vi "读取CODMn数据波形新.vi"() -> ()   [LabVIEW 2016, in "斯坦道CODMn新电路板.lvlib"]
uses:
  <vilib>/Utility/miscctls.llb/LVPointTypeDef.ctl
  <userlib>/_OpenG.lib/array/array.llb/Sort 1D Array (I32)__ogtk.vi
  <vilib>/Waveform/WDTFileIO.llb/Read Waveform from File.vi
panel:
  in  "页":i32 format="第%.0f页"
  in  "每页条数":i32=20
  in  "向后按钮":bool
  in  "向前按钮":bool
  in  "数据表":T1
  in  "查看曲线数组":bool[](array[boolean])
  in  "打开波形文件":bool
  in  "簇":cluster{"数据起始时间":timestamp, "数据终止时间":timestamp}
  in  "查询":bool
  in  "当前滴定曲线":bool
  in  "当前温度曲线":bool
  in  "关闭":bool
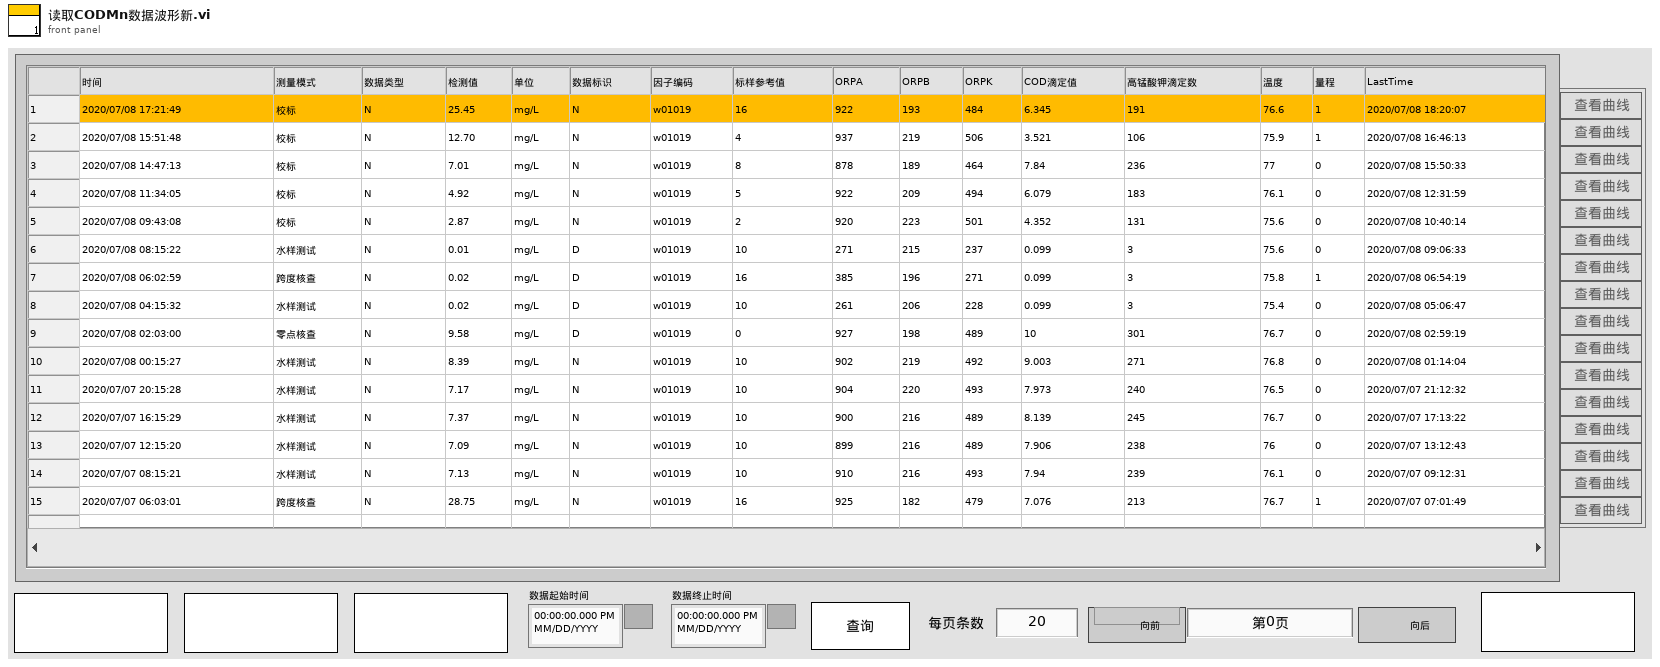
[diagram p1: front panel]
types:
  T1 = typedef "数据查询大列表框.ctl" = i32
  T2 = typedef "LVPointTypeDef.ctl" = cluster{"Horizontal":i16, "Vertical":i16}
  T3 = cluster{timestamp, "seconds since 1Jan1904":timestamp}
  T4 = enum16{"Left Button", "Center Button", "Right Button", "Window Close"}
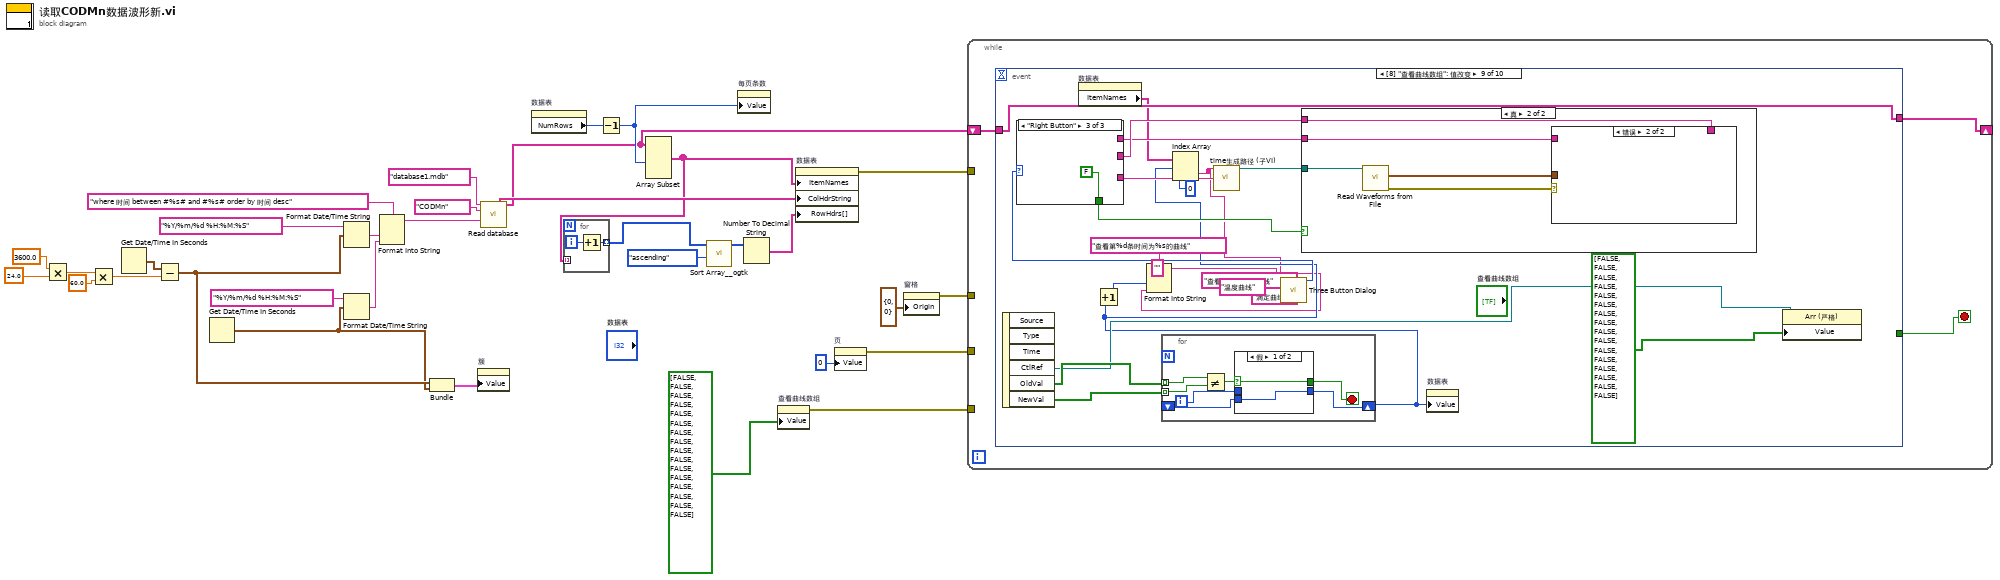
[diagram p0: block diagram]
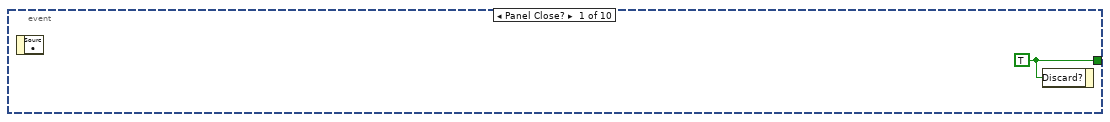
[diagram p2: hidden frame]
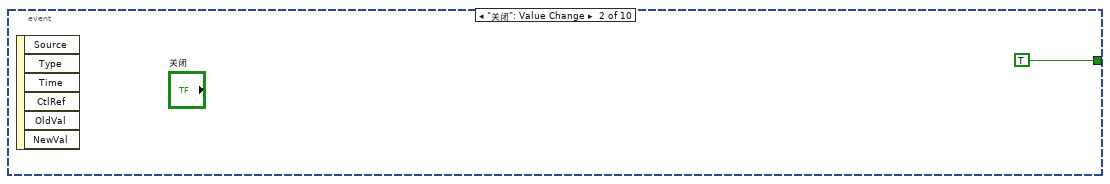
[diagram p3: hidden frame]
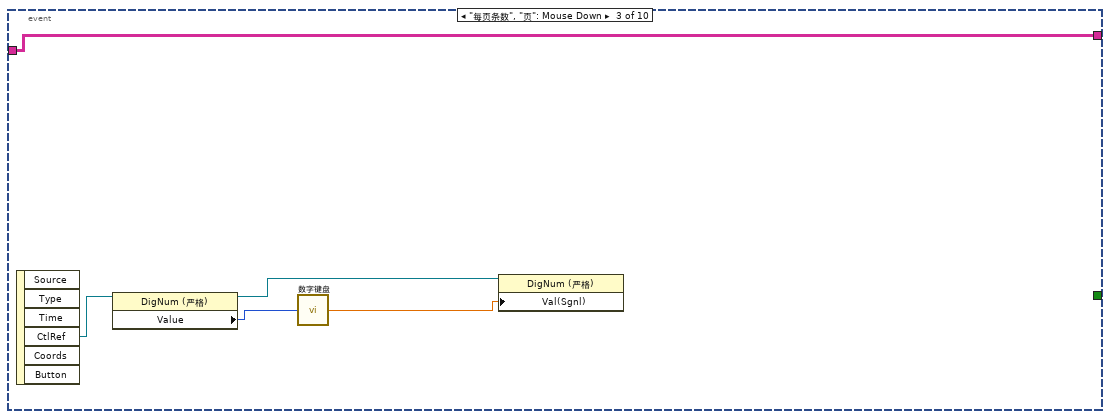
[diagram p4: hidden frame]
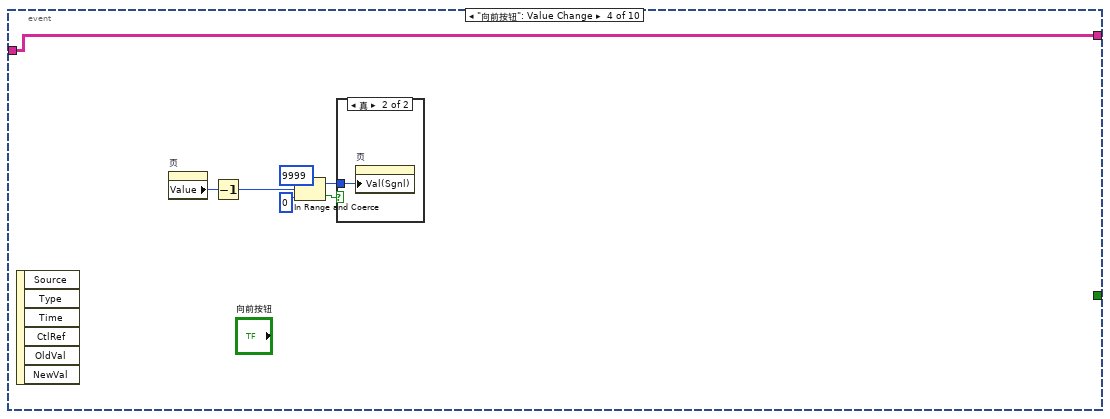
[diagram p5: hidden frame]
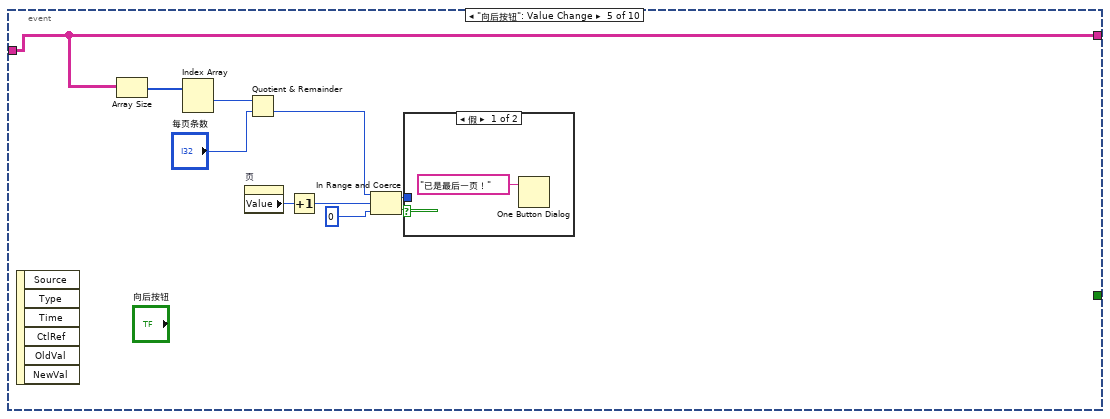
[diagram p7: hidden frame]
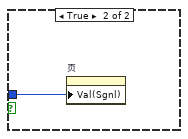
[diagram p8: hidden frame]
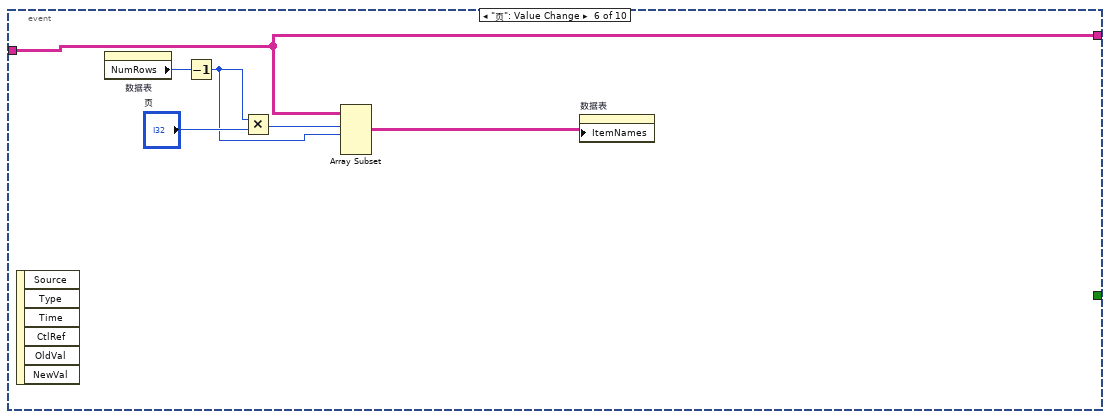
[diagram p9: hidden frame]
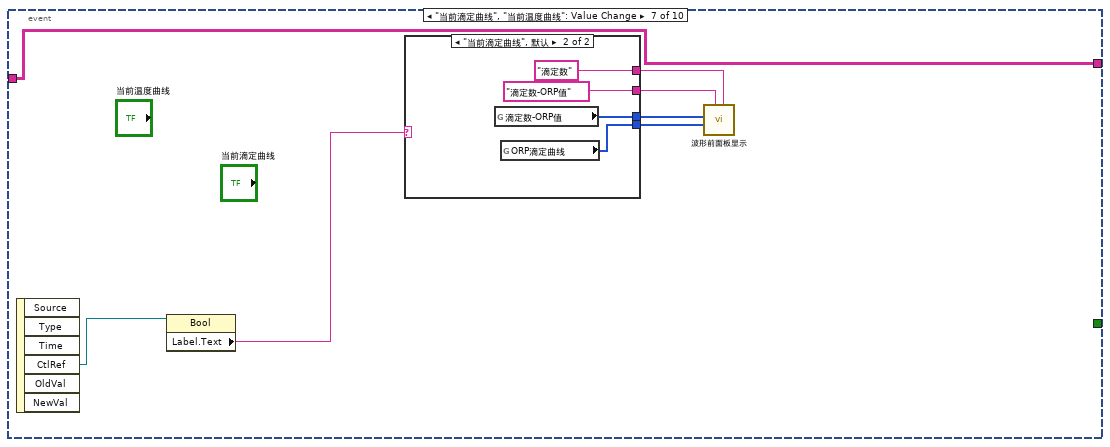
[diagram p10: hidden frame]
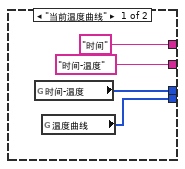
[diagram p11: hidden frame]
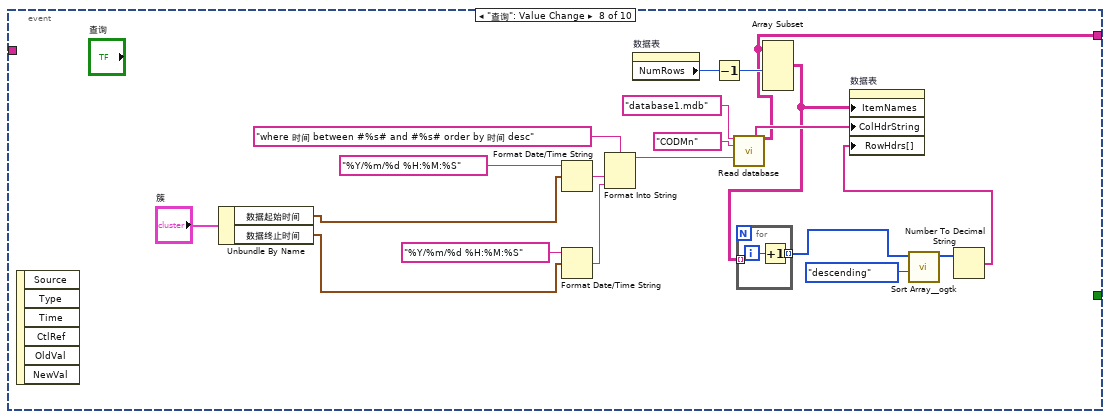
[diagram p12: hidden frame]
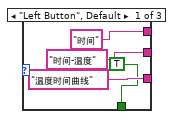
[diagram p14: hidden frame]
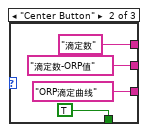
[diagram p15: hidden frame]
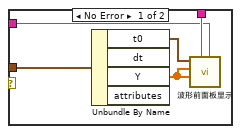
[diagram p17: hidden frame]
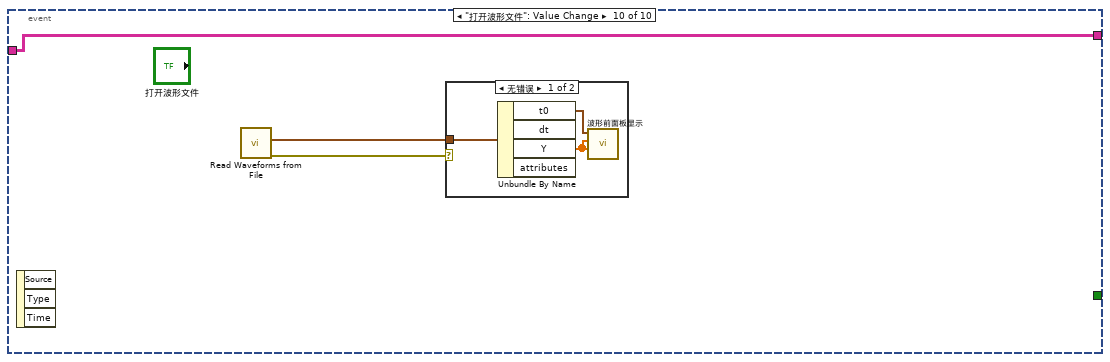
[diagram p18: hidden frame]
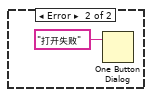
[diagram p19: hidden frame]
diagram:
  n1 = Multiply(x=3600.0, y=24.0) -> (x*y=w30:dbl)
  n2 = Multiply(x=w30, y=60.0) -> (x*y=w28:dbl)
  n3 = Get Date/Time In Seconds() -> (seconds since 1Jan1904=w33:timestamp)
  n4 = Subtract(x=w33, y=w28) -> (x-y=w3:timestamp)
  n5 = Get Date/Time In Seconds() -> (seconds since 1Jan1904=w2:timestamp)
  n6 = Format Date/Time String(time format string (%c)="%Y/%m/%d %H:%M:%S" ("时间格式字符串(%c)"), seconds (now)=w3) -> (date/time string=w25:string)  [unwired: 1 in]
  n7 = Format Date/Time String(time format string (%c)="%Y/%m/%d %H:%M:%S" ("时间格式字符串(%c)"), seconds (now)=w2) -> (date/time string=w26:string)  [unwired: 1 in]
  n8 = Format Into String(format string="where 时间 between #%s# and #%s# order by 时间 desc" ("condition"), w25, w26) -> (resulting string=w27:string)  [unwired: 2 in, 1 out]
  n9 = Bundle(w3, "seconds since 1Jan1904"=w2) -> (w1:T3)  [unwired: 1 in]
  n10 = property on="簇" class="Clust (严格)"("Value"=w1) -> ()  [unwired: 2 in, 2 out]
  n11 = call "Read database.vi"("database"="database1.mdb", "组合框"="CODMn", "condition"=w27) -> ("columns"=w19:string[], "表格"=w10:string[][])  [unwired: 7 in, 4 out]
  n12 = property on="数据表" class="MCListbox (严格)"() -> ("NumRows"=w13:u32)  [unwired: 2 in, 2 out]
  n13 = Decrement(x=w13) -> (x-1=w11:u32)
  n14 = Array Subset(array=w10, length (row)=w11) -> (w12:string[][])  [unwired: 3 in]
  n15 = for {
    tunnel: [w34] -> w18 mode=indexing
    tunnel: w12 -> [_] mode=indexing
    i -> [w35]
    n16 = Increment(x=w35) -> (x+1=w34:i32)
  }
  n17 = call-poly <userlib>:"Sort Array__ogtk.vi"("Order"=enum16{"ascending", "descending"}."ascending", "Array in"=w18) -> ("Sorted Array out"=w16:i32[])  [unwired: 8 in, 1 out]
  n18 = property on="每页条数" class="DigNum (严格)"("Value"=w11) -> ()  [unwired: 2 in, 2 out]
  n19 = Number To Decimal String(number=w16) -> (decimal integer string=w15:string[])  [unwired: 1 in]
  n20 = property on="查看曲线数组" class="Arr (严格)"("Value"=bool[] [FALSE, FALSE, FALSE, FALSE, FALSE, FALSE, FALSE, FALSE, FALSE, FALSE, FALSE, FALSE, FALSE, FALSE, FALSE, FALSE] ("查看曲线数组")) -> (error out=w4:errorcluster)  [unwired: 2 in, 1 out]
  n21 = property on="数据表" class="MCListbox (严格)"("ItemNames"=w12, "ColHdrString"=w19, "RowHdrs[]"=w15) -> (error out=w14:errorcluster)  [unwired: 2 in, 1 out]
  n22 = property on="页" class="DigNum (严格)"("Value"=0 ("页")) -> (error out=w8:errorcluster)  [unwired: 2 in, 1 out]
  n23 = property on="窗格" class="Pane"("Origin"=T2 {"Horizontal"=0, "Vertical"=0} ("原点")) -> (error out=w6:errorcluster)  [unwired: 2 in, 1 out]
  n24 = while {
    tunnel: w14 -> [_]
    shift-right: [w36] -> _
    shift-left: w10 -> [w37]
    tunnel: w8 -> [_]
    tunnel: w6 -> [_]
    tunnel: w4 -> [_]
    stop <- w38 stop-if-true
    n25 = event shown="[8] \"查看曲线数组\": 值改变" {
      selector: _ -> [_ _ _ _ _ _ _ _ _ _]
      dyn-events: _ -> [_ _ _ _ _ _ _ _ _ _]
      timeout: _ -> [_ _ _ _ _ _ _ _ _ _]
      tunnel: [w39 TRUE ("Discard?") _ _ _ _ _ _ _ _] -> w38
      tunnel: w37 -> [_ _ w41 w46 w58 w66 w72 _ w113 w160]
      tunnel: [_ _ w41 w46 w58 w66 w72 w87 w113 w160] -> w36
      event Panel Close? {
        w39 = TRUE ("Discard?")
        n26 = event-data() -> ()  [unwired: 1 in, 1 out]
        n27 = event-data("Discard?"=w39) -> ()  [unwired: 1 in, 1 out]
      }
      event "关闭": Value Change {
        n28 = event-data() -> ()  [unwired: 1 in, 6 out]
      }
      event "每页条数", "页": Mouse Down {
        n29 = event-data() -> ("CtlRef"=w45:refnum<vi>)  [unwired: 1 in, 5 out]
        n30 = property class="DigNum (严格)"(reference=w45) -> (reference out=w43:refnum<vi>, "Value"=w44:i32)  [unwired: 1 in, 1 out]
        n31 = call "数字键盘.vi"("OldNumber"=w44) -> ("NewNumber"=w42:dbl)
        n32 = property class="DigNum (严格)"(reference=w43, "Val(Sgnl)"=w42) -> ()  [unwired: 1 in, 2 out]
      }
      event "向前按钮": Value Change {
        n33 = event-data() -> ()  [unwired: 1 in, 6 out]
        n34 = property on="页" class="DigNum (严格)"() -> ("Value"=w47:i32)  [unwired: 2 in, 2 out]
        n35 = Decrement(x=w47) -> (x-1=w52:i32)
        n36 = In Range and Coerce(upper limit=9999 ("上限"), x=w52, lower limit=0 ("下限")) -> (coerced(x)=w49:i32, In Range?=w48:bool)
        n37 = case shown="真" w48 {
          tunnel: w49 -> [_ w53]
          frame False {
          }
          frame True {
            n38 = property on="页" class="DigNum (严格)"("Val(Sgnl)"=w53) -> ()  [unwired: 2 in, 2 out]
          }
        }
      }
      event "向后按钮": Value Change {
        n39 = event-data() -> ()  [unwired: 1 in, 6 out]
        n40 = Array Size(array=w58) -> (size(s)=w57:i32[])
        n41 = Index Array(array=w57) -> (element #1=w56:i32)  [unwired: 2 in, 1 out]
        n42 = property on="页" class="DigNum (严格)"() -> ("Value"=w59:i32)  [unwired: 2 in, 2 out]
        n43 = Quotient & Remainder(x=w56, y="每页条数") -> (floor(x/y)=w54:i32)  [unwired: 1 out]
        n44 = Increment(x=w59) -> (x+1=w63:i32)
        n45 = In Range and Coerce(upper limit=w54, x=w63, lower limit=0 ("下限")) -> (coerced(x)=w61:i32, In Range?=w60:bool)
        n46 = case shown="假" w60 {
          tunnel: w61 -> [_ w65]
          frame False {
            n47 = One Button Dialog(message="已是最后一页！" ("消息")) -> ()  [unwired: 1 in, 1 out]
          }
          frame True {
            n48 = property on="页" class="DigNum (严格)"("Val(Sgnl)"=w65) -> ()  [unwired: 2 in, 2 out]
          }
        }
      }
      event "页": Value Change {
        n49 = event-data() -> ()  [unwired: 1 in, 6 out]
        n50 = property on="数据表" class="MCListbox (严格)"() -> ("NumRows"=w70:u32)  [unwired: 2 in, 2 out]
        n51 = Decrement(x=w70) -> (x-1=w68:u32)
        n52 = Multiply(x=w68, y="页") -> (x*y=w69:u32)
        n53 = Array Subset(array=w66, index (row)=w69, length (row)=w68) -> (w67:string[][])  [unwired: 2 in]
        n54 = property on="数据表" class="MCListbox (严格)"("ItemNames"=w67) -> ()  [unwired: 2 in, 2 out]
      }
      event "当前滴定曲线", "当前温度曲线": Value Change {
        n55 = event-data() -> ("CtlRef"=w76:refnum<vi>)  [unwired: 1 in, 5 out]
        n56 = property class="Bool"(reference=w76) -> ("Label.Text"=w75:string)  [unwired: 1 in, 2 out]
        n57 = case shown="\"当前滴定曲线\", 默认" w75 {
          tunnel: [w81 w86] -> w78
          tunnel: [w82 w85] -> w77
          tunnel: ["时间-温度" ("标题.文本") "滴定数-ORP值" ("标题.文本")] -> w74
          tunnel: ["时间" ("X标尺.名称标签.文本") "滴定数" ("X标尺.名称标签.文本")] -> w73
          frame "当前温度曲线" {
            n58 = global read "VARCODMn全局变量.vi" "时间-温度"() -> (w82:u16[])
            n59 = global read "VARCODMn全局变量.vi" "温度曲线"() -> (w81:u16[])
          }
          frame "当前滴定曲线", Default {
            n60 = global read "VARCODMn全局变量.vi" "滴定数-ORP值"() -> (w85:u16[])
            n61 = global read "VARCODMn全局变量.vi" "ORP滴定曲线"() -> (w86:u16[])
          }
        }
        n62 = call "波形前面板显示.vi"("X标尺.名称标签.文本"=w73, "标题.文本"=w74, "ORP滴定曲线"=w78, "滴定数-ORP值"=w77) -> ()  [unwired: 8 in]
      }
      event "查询": Value Change {
        n63 = event-data() -> ()  [unwired: 1 in, 6 out]
        n64 = Unbundle By Name("簇") -> ("数据起始时间"=w98:timestamp, "数据终止时间"=w97:timestamp)
        n65 = Format Date/Time String(time format string (%c)="%Y/%m/%d %H:%M:%S" ("时间格式字符串(%c)"), seconds (now)=w98) -> (date/time string=w102:string)  [unwired: 1 in]
        n66 = Format Date/Time String(time format string (%c)="%Y/%m/%d %H:%M:%S" ("时间格式字符串(%c)"), seconds (now)=w97) -> (date/time string=w103:string)  [unwired: 1 in]
        n67 = Format Into String(format string="where 时间 between #%s# and #%s# order by 时间 desc" ("condition"), w102, w103) -> (resulting string=w96:string)  [unwired: 2 in, 1 out]
        n68 = property on="数据表" class="MCListbox (严格)"() -> ("NumRows"=w89:u32)  [unwired: 2 in, 2 out]
        n69 = Decrement(x=w89) -> (x-1=w90:u32)
        n70 = call "Read database.vi"("database"="database1.mdb", "组合框"="CODMn", "condition"=w96) -> ("columns"=w95:string[], "表格"=w87:string[][])  [unwired: 7 in, 4 out]
        n71 = Array Subset(array=w87, length (row)=w90) -> (w88:string[][])  [unwired: 3 in]
        n72 = for {
          tunnel: [w107] -> w94 mode=indexing
          tunnel: w88 -> [_] mode=indexing
          i -> [w108]
          n73 = Increment(x=w108) -> (x+1=w107:i32)
        }
        n74 = call-poly <userlib>:"Sort Array__ogtk.vi"("Order"=enum16{"ascending", "descending"}."descending", "Array in"=w94) -> ("Sorted Array out"=w92:i32[])  [unwired: 8 in, 1 out]
        n75 = Number To Decimal String(number=w92) -> (decimal integer string=w91:string[])  [unwired: 1 in]
        n76 = property on="数据表" class="MCListbox (严格)"("ItemNames"=w88, "ColHdrString"=w95, "RowHdrs[]"=w91) -> ()  [unwired: 2 in, 2 out]
      }
      event "查看曲线数组": Value Change {
        (unwired) "查看温度或滴定曲线" ("message")
        n77 = event-data() -> ("CtlRef"=w119:refnum<vi>, "OldVal"=w121:bool[], "NewVal"=w120:bool[])  [unwired: 1 in, 3 out]
        n78 = property on="数据表" class="MCListbox (严格)"() -> ("ItemNames"=w109:string[][])  [unwired: 2 in, 2 out]
        n79 = for {
          tunnel: w121 -> [w136] mode=indexing
          tunnel: w120 -> [w135] mode=indexing
          shift-right: [w132] -> w112
          shift-left: _ -> [w131]
          i -> [w133]
          stop <- w130 stop-if-true
          n80 = Not Equal?(x=w136, y=w135) -> (x != y?=w134:bool)
          n81 = case shown="假" w134 {
            selector: w134 -> [w138 w139]
            tunnel: w133 -> [_ w140]
            tunnel: [w137 w140] -> w132
            tunnel: [w138 w139] -> w130
            tunnel: w131 -> [w137 _]
            frame False {
            }
            frame True {
            }
          }
        }
        n82 = Increment(x=w112) -> (x+1=w114:i32)
        n83 = Index Array(array=w109, index (row)=w112, index (col)=0 ("长度")) -> (element=w110:string)
        n84 = Format Into String(format string="查看第%d条时间为%s的曲线" ("格式字符串"), initial string="" ("初始字符串"), w114, w110) -> (resulting string=w115:string)  [unwired: 1 in, 1 out]
        n85 = call <vilib>:"Three Button Dialog.vi"("Center Button Text (\"No\")"="滴定曲线" ("Center Button Text (\"No\")"), "Left Button Text (\"Yes\")"="温度曲线" ("Left Button Text (\"Yes\")"), "message"=w115) -> ("Which Button?"=w123:T4)  [unwired: 8 in]
        n86 = case shown="\"Right Button\"" w123 {
          tunnel: ["温度时间曲线" ("名称或相对路径") "ORP滴定曲线" ("名称或相对路径") _] -> w128
          tunnel: ["时间-温度" ("标题.文本") "滴定数-ORP值" ("标题.文本") _] -> w127
          tunnel: ["时间" ("X标尺.名称标签.文本") "滴定数" ("X标尺.名称标签.文本") _] -> w126
          tunnel: [TRUE TRUE FALSE] -> w122
          frame "Left Button", Default {
          }
          frame "Center Button" {
          }
          frame "Right Button" {
          }
        }
        n87 = call "time生成路径 (子VI).vi"("名称或相对路径"=w128, "时间"=w110) -> ("appended path"=w129:path)  [unwired: 9 in]
        n88 = case shown="真" w122 {
          tunnel: w129 -> [_ w152]
          tunnel: w127 -> [_ w151]
          tunnel: w126 -> [_ w150]
          frame False {
          }
          frame True {
            n89 = call-poly <vilib>:"Read Waveforms from File.vi"("file path (dialog if empty)"=w152) -> ("error out"=w154:errorcluster, "first waveform in record"=w153:waveform(dbl))  [unwired: 5 in, 2 out]
            n90 = case shown="错误" w154 {
              tunnel: w153 -> [w159 _]
              tunnel: w151 -> [w156 _]
              tunnel: w150 -> [w155 _]
              frame No Error {
                n91 = Unbundle By Name(w159) -> ("t0"=w158:timestamp, "Y"=w157:dbl[])  [unwired: 2 out]
                n92 = call "波形前面板显示.vi"("X标尺.名称标签.文本"=w155, "标题.文本"=w156, "ORP滴定曲线"=w157, "滴定数-ORP值"=w157, "波形时间"=w158) -> ()  [unwired: 7 in]
              }
              frame Error {
              }
            }
          }
        }
        n93 = property on="数据表" class="MCListbox (严格)"("Value"=w112) -> ()  [unwired: 2 in, 2 out]
        n94 = property class="Arr (严格)"(reference=w119, "Value"=bool[] [FALSE, FALSE, FALSE, FALSE, FALSE, FALSE, FALSE, FALSE, FALSE, FALSE, FALSE, FALSE, FALSE, FALSE, FALSE, FALSE] ("查看曲线数组")) -> ()  [unwired: 1 in, 2 out]
      }
      event "打开波形文件": Value Change {
        n95 = event-data() -> ()  [unwired: 1 in, 3 out]
        n96 = call-poly <vilib>:"Read Waveforms from File.vi"() -> ("error out"=w162:errorcluster, "first waveform in record"=w161:waveform(dbl))  [unwired: 6 in, 2 out]
        n97 = case shown="无错误" w162 {
          tunnel: w161 -> [w165 _]
          frame No Error {
            n98 = Unbundle By Name(w165) -> ("t0"=w164:timestamp, "Y"=w163:dbl[])  [unwired: 2 out]
            n99 = call "波形前面板显示.vi"("ORP滴定曲线"=w163, "滴定数-ORP值"=w163, "波形时间"=w164) -> ()  [unwired: 9 in]
          }
          frame Error {
            n100 = One Button Dialog(message="打开失败" ("消息")) -> ()  [unwired: 1 in, 1 out]
          }
        }
      }
    }
  }
